vi "THETA_2.vi"(8 "error in (no error)":errorcluster, 11 "reference in":refnum<class "Manipulator.lvclass">) -> (0 "error out":errorcluster, 3 "reference out":refnum<class "Manipulator.lvclass">)   [LabVIEW 2014, in "Manipulator.lvclass"]
uses:
  Manipulator.lvclass
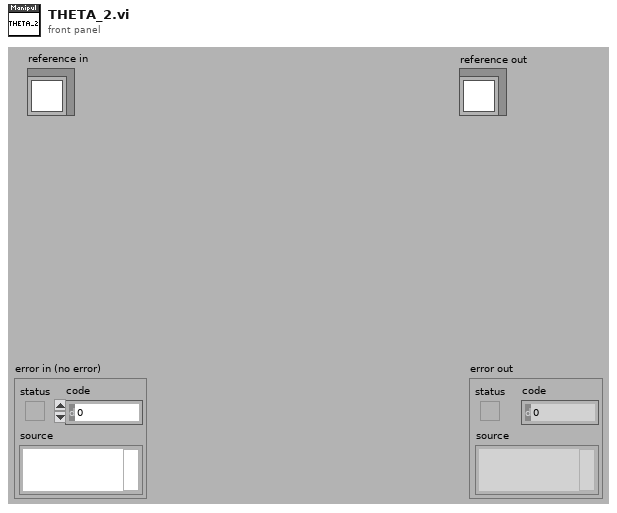
[diagram p1: front panel]
types:
  T1 = typedef "Manipulator.lvclass/ObjectAttributes.ctl" = cluster{"Coordinates":cluster{"X":dbl, "Y":dbl, "Z":dbl}, "Angles":cluster{"THETA_1":dbl, "THETA_2":dbl, "THETA_3":dbl, "THETA_4":dbl, "THETA_5":dbl, "THETA_6":dbl, "THETA_7":dbl, "THETA_8":dbl, "THETA_9":dbl, "THETA_10":dbl}, "Lengths":cluster{"a":dbl, "b":dbl, "c":dbl, "d":dbl, "e":dbl}, "Coordinates of joints":cluster{"A":cluster{"X":dbl, "Y":dbl, "Z":dbl}, "B":cluster{"X":dbl, "Y":dbl, "Z":dbl}, "C":cluster{"X":dbl, "Y":dbl, "Z":dbl}, "D":cluster{"X":dbl, "Y":dbl, "Z":dbl}}}
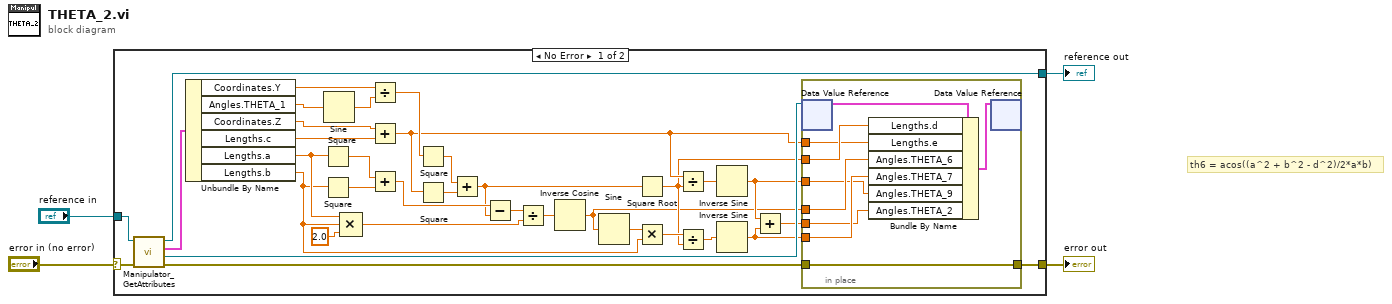
[diagram p0: block diagram]
diagram:
  # "th6 = acos((a^2 + b^2 - d^2)/2*a*b)"
  n1 = case shown="No Error" "error in (no error)" {
    selector: "error in (no error)" -> [w38 w50]
    tunnel: [w13 w50] -> w3
    tunnel: [w5 w49] -> w1
    tunnel: "reference in" -> [w39 w49]
    frame No Error {
      n2 = call "Manipulator_GetAttributes.vi"("error in (no error)"=w38, "reference in"=w39) -> ("error out"=w35:errorcluster, "DataRef"=w36:refnum<data-value>, "Data"=w37:T1, "reference out"=w5:refnum<class "Manipulator.lvclass">)  [unwired: 6 in]
      n3 = Unbundle By Name(w37) -> ("Coordinates.Y"=w34:dbl, "Angles.THETA_1"=w28:dbl, "Coordinates.Z"=w32:dbl, "Lengths.c"=w27:dbl, "Lengths.a"=w21:dbl, "Lengths.b"=w16:dbl)
      n4 = Square(x=w21) -> (x^2=w26:dbl)
      n5 = Square(x=w16) -> (x^2=w25:dbl)
      n6 = Sine(x=w28) -> (sin(x)=w33:dbl)
      n7 = Compound Arithmetic op=MULTIPLY(w21, w16, 2.0 ("value")) -> (w19:dbl)
      n8 = Divide(x=w34, y=w33) -> (x/y=w29:dbl)
      n9 = Add(x=w32, y=w27) -> (x+y=w11:dbl)
      n10 = Add(x=w26, y=w25) -> (x+y=w24:dbl)
      n11 = Square(x=w29) -> (x^2=w31:dbl)
      n12 = Square(x=w11) -> (x^2=w30:dbl)
      n13 = Add(x=w31, y=w30) -> (x+y=w23:dbl)
      n14 = Subtract(x=w24, y=w23) -> (x-y=w22:dbl)
      n15 = Divide(x=w22, y=w19) -> (x/y=w18:dbl)
      n16 = Inverse Cosine(1:w18) -> (0:w6:dbl)
      n17 = Sine(x=w6) -> (sin(x)=w17:dbl)
      n18 = Square Root(x=w23) -> (sqrt(x)=w10:dbl)
      n19 = Multiply(x=w17, y=w16) -> (x*y=w15:dbl)
      n20 = Divide(x=w11, y=w10) -> (x/y=w12:dbl)
      n21 = Divide(x=w15, y=w10) -> (x/y=w14:dbl)
      n22 = Inverse Sine(1:w12) -> (0:w8:dbl)
      n23 = Inverse Sine(1:w14) -> (0:w9:dbl)
      n24 = Add(x=w8, y=w9) -> (x+y=w7:dbl)
      n25 = in-place {
        in-place-border: w35 -> [w48]
        in-place-border: [w48] -> w13
        in-place-border: w10 -> [w45]
        in-place-border: w11 -> [w44]
        in-place-border: w6 -> [w43]
        in-place-border: w9 -> [w42]
        in-place-border: w8 -> [w41]
        in-place-border: w7 -> [w40]
        n26 = in-place-dvr #1(w36) -> (w46:T1)  [unwired: 1 out]
        n27 = Bundle By Name(cluster=w46, "Lengths.d"=w45, "Lengths.e"=w44, "Angles.THETA_6"=w43, "Angles.THETA_7"=w42, "Angles.THETA_9"=w41, "Angles.THETA_2"=w40) -> (w47:T1)
        n28 = in-place-dvr #1(w47) -> ()  [unwired: 2 out]
      }
    }
    frame Error {
    }
  }
  "error out" <- w3
  "reference out" <- w1
